vi "Errors.vi"   [LabVIEW 2019, in "DSF Core.lvlib" / "Buffer.lvclass"]
doc: "Polymorphic VI that throws Buffer errors."
uses:
  Buffer.lvclass
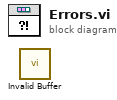
[diagram p0: block diagram]
diagram:
  n1 = call "Invalid Buffer.vi"() -> ()  [unwired: 10 in, 2 out]
